vi "Write Numeric.vi"(8 "error in (no error)":errorcluster, 10 "Numeric":i64, 11 "Product-A in":refnum<class "Product-A.lvclass">) -> (0 "error out":errorcluster, 3 "Product-A out":refnum<class "Product-A.lvclass">)   [LabVIEW 2018, in "Product-A.lvclass"]
uses:
  Product-A.lvclass
  Product-A.lvclass/Product-A.ctl
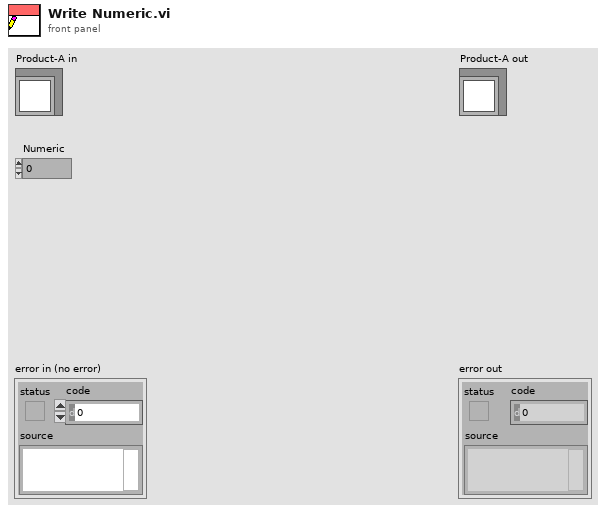
[diagram p1: front panel]
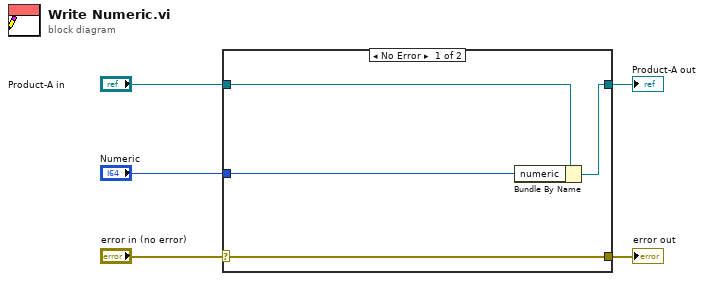
[diagram p0: block diagram]
diagram:
  n1 = case shown="No Error" "error in (no error)" {
    selector: "error in (no error)" -> [w9 w10]
    tunnel: [w9 w10] -> w4
    tunnel: [w7 w11] -> w2
    tunnel: "Product-A in" -> [w8 w11]
    tunnel: "Numeric" -> [w6 _]
    frame No Error {
      n2 = Bundle By Name(cluster=w8, "numeric"=w6) -> (w7:refnum<class "Product-A.lvclass">)
    }
    frame Error {
    }
  }
  "error out" <- w4
  "Product-A out" <- w2
